vi "Alpha Ver 2.2.vi"() -> ()   [LabVIEW 2015]
uses:
  <instrlib>/Keithley 622x LV 2009/Keithley 622x.lvlib
  <instrlib>/Keithley 622x LV 2009/Utility/Typedefs/KE622x -- Instrument Type.ctl
panel:
  out "Measurements":string
  in  "Comments":string
  out "FILE":refnum<file>
  in  "Folder \nPrename":string
  out "Output command string":string
  out "Example of commands":string="*RST\nSOUR:PDEL:HIGH 1e-3\nSOUR:PDEL:LOW 0\nSOUR:PDEL:WIDT 500e-6\nSOUR:PDEL:SDEL 100e-6\nSOUR:PDEL:COUN INF\nSOUR:PDEL:RANG BEST\nSOUR:PDEL:INT 5\nSOUR:PDEL:LME 2\nTRAC:POIN 200\nSOUR:PDEL:ARM\nINIT:IMM"
  out "LM_com":string
  out "I_com":string
  out "R_com":string
  out "C_com":string
  out "SD_com":string
  out "W_com":string
  out "LL_com":string
  out "HL_com":string
  in  "INF Button":bool
  in  "prefix 2":u16(ring)
  in  "prefix":u16(ring)
  in  "Low Measure":u16(ring)=1 items=["1", "2"]
  in  "Interval":dbl=5.0 min=5.0 max=999999.0 step=1.0
  in  "Ranging":string(combo)="BEST"
  in  "Count":dbl=1.0 min=1.0 max=65536.0 step=1.0
  in  "Source Delay":dbl
  in  "Width":dbl
  in  "Low Level":dbl min=-0.105 max=0.105
  in  "High Level":dbl
  out "2182A \nconnected ?":string
  in  "STOP":bool
  out "Measurement\nUnits":string
  out "2182A Voltage \nRange":string
  out "error out":errorcluster
  # "Pulse Measurement System"
  # "SYSTEM INFORMATION"
  # "FILE CONFIGURATION"
  # "PULSE SETTINGS"
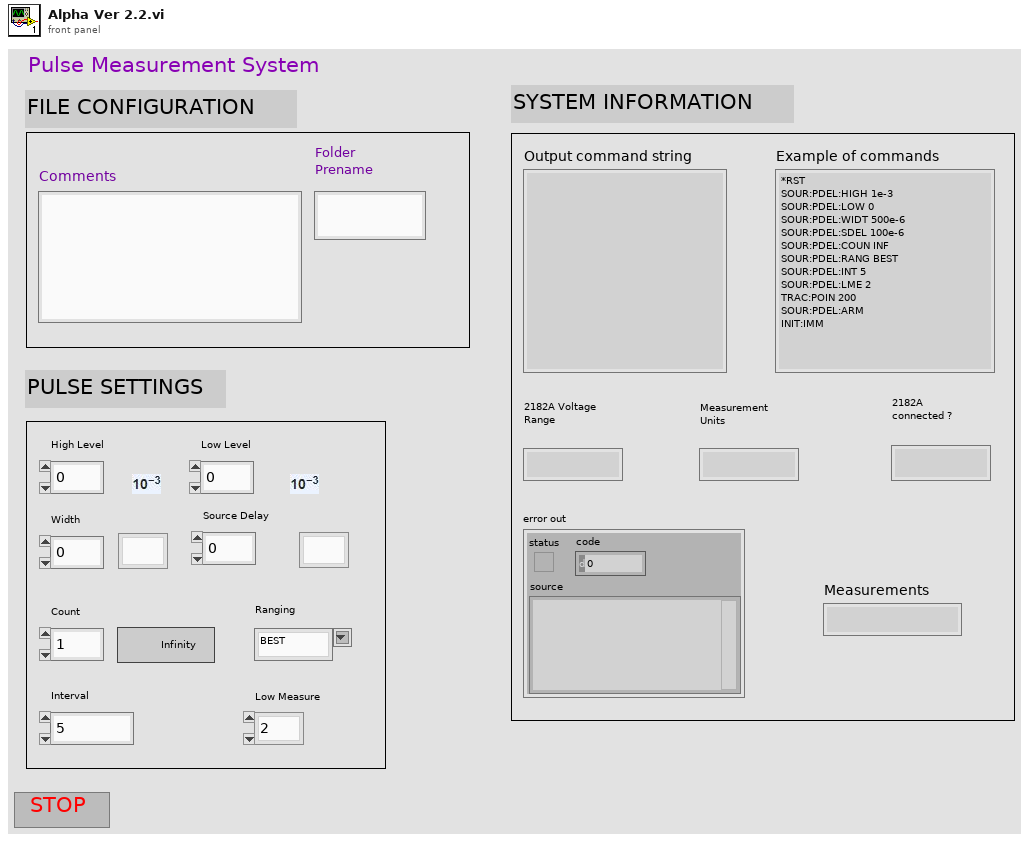
[diagram p1: front panel]
types:
  T1 = typedef "Keithley 622x.lvlib/KE622x -- Instrument Type.ctl" = enum16{"KE6220", "KE6221"}
  T2 = cluster{"VISA resource name out":refnum<visa-resource-name>, "error out":errorcluster}
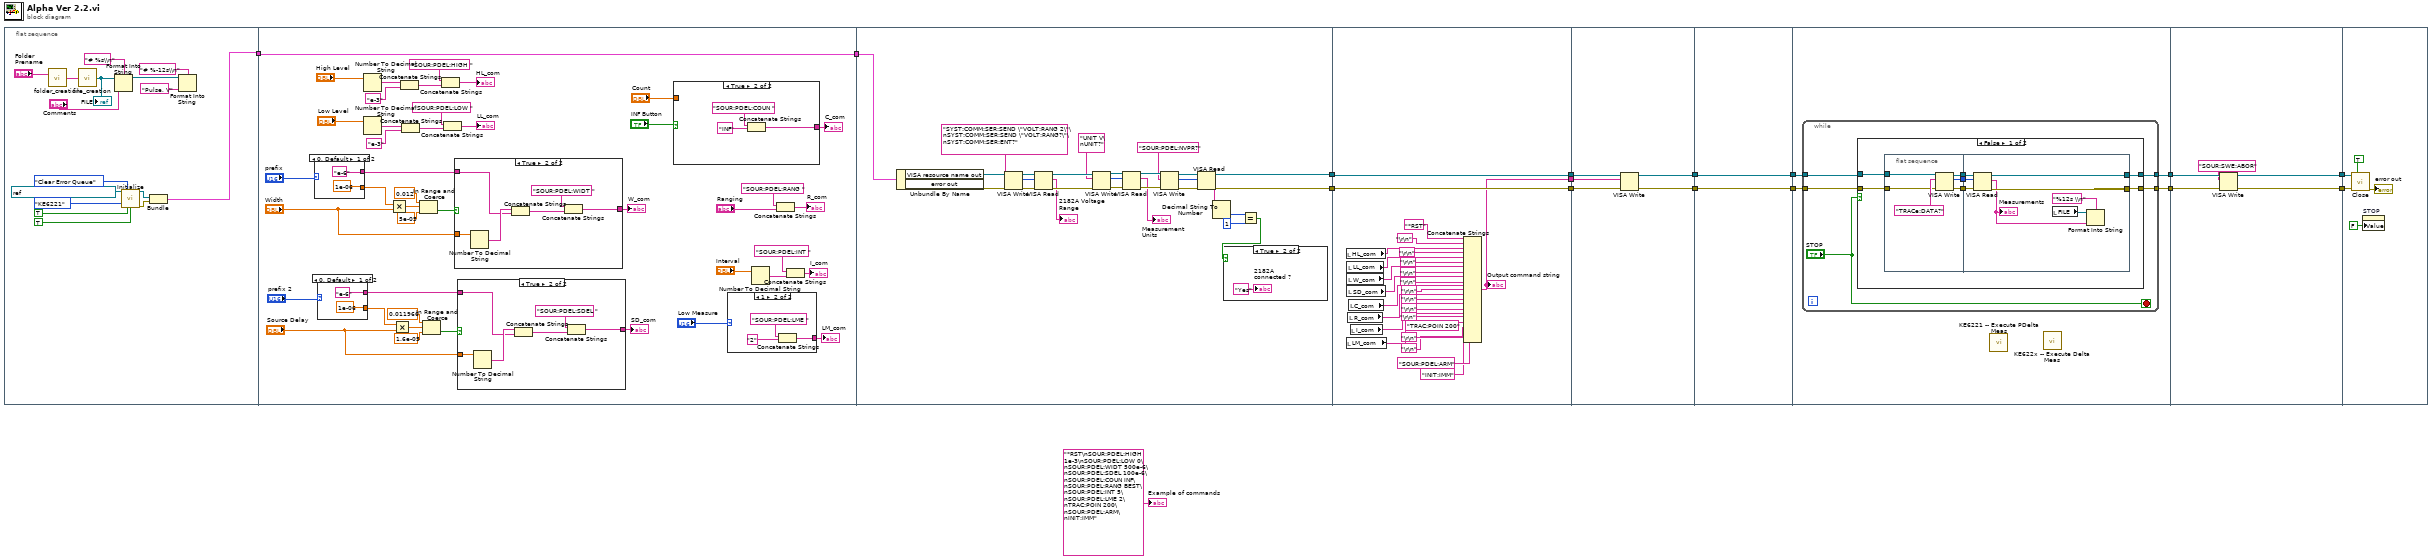
[diagram p0: block diagram]
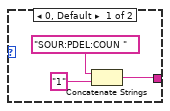
[diagram p2: hidden frame]
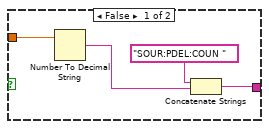
[diagram p3: hidden frame]
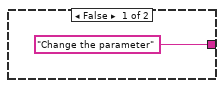
[diagram p4: hidden frame]
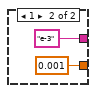
[diagram p5: hidden frame]
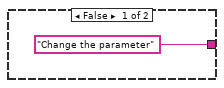
[diagram p6: hidden frame]
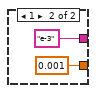
[diagram p7: hidden frame]
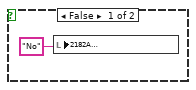
[diagram p8: hidden frame]
diagram:
  n1 = flat-sequence {
    tunnel: [w25] -> w16
    tunnel: w16 -> [w33]
    tunnel: [w33] -> w15
    tunnel: [w115] -> w14
    tunnel: [w114] -> w12
    tunnel: w15 -> [w113]
    tunnel: w14 -> [w165]
    tunnel: [w165] -> w13
    tunnel: w12 -> [w164]
    tunnel: [w164] -> w11
    tunnel: [w144] -> w9
    tunnel: w13 -> [w170]
    tunnel: [w169] -> w8
    tunnel: w11 -> [w168]
    tunnel: [w167] -> w6
    tunnel: w9 -> [w166]
    tunnel: w8 -> [w172]
    tunnel: [w172] -> w7
    tunnel: w6 -> [w171]
    tunnel: [w171] -> w5
    tunnel: w7 -> [w176]
    tunnel: w5 -> [w175]
    tunnel: [w174] -> w4
    tunnel: [w173] -> w2
    tunnel: w4 -> [w209]
    tunnel: [w208] -> w3
    tunnel: w2 -> [w207]
    tunnel: [w206] -> w1
    tunnel: w3 -> [w212]
    tunnel: w1 -> [w211]
    frame #0 {
      n2 = call "folder_creation.vi"("Name"="Folder \nPrename") -> ("String"=w23:string)
      n3 = call "file_creation.vi"("String"=w23) -> ("refnum out"=w22:refnum<file>)
      "FILE" <- w22
      n4 = Format Into String(format string="# %s\\n", initial string=w22, "Comments") -> (resulting string=w17:refnum<file>)  [unwired: 1 in, 1 out]
      n5 = call <instrlib>:"Initialize.vi"("VISA resource name"=refnum<visa-resource-name> "DC_AC_Current_Source_6221", "Error Queue Option"=enum16{"Clear Error Queue", "Error Query"}."Clear Error Queue", "Instrument Type"=KE622x_--_Instrument_Type."KE6221", "ID Query? (T)"=TRUE, "Reset? (T)"=TRUE) -> ("VISA resource name out"=w27:refnum<visa-resource-name>, "error out"=w26:errorcluster)  [unwired: 9 in]
      n6 = Bundle("VISA resource name out"=w27, "error out"=w26) -> (w25:T2)  [unwired: 1 in]
      n7 = Format Into String(format string="# %-12s\\n", initial string=w17, "Pulse, V" ("input 3")) -> ()  [unwired: 1 in, 2 out]
    }
    frame #1 {
      n8 = case shown="0, Default" "prefix" {
        tunnel: [1e-06 0.001] -> w56
        tunnel: ["e-6" ("string") "e-3" ("string")] -> w61
        frame 0, Default {
        }
        frame 1 {
        }
      }
      n9 = case shown="0, Default" "prefix 2" {
        tunnel: [1e-06 0.001] -> w51
        tunnel: ["e-6" ("string") "e-3" ("string")] -> w46
        frame 0, Default {
        }
        frame 1 {
        }
      }
      n10 = Number To Decimal String(number="High Level") -> (decimal integer string=w72:string)  [unwired: 1 in]
      n11 = Number To Decimal String(number="Low Level") -> (decimal integer string=w67:string)  [unwired: 1 in]
      n12 = Multiply(x=w56, y="Width") -> (x*y=w57:dbl)
      n13 = Multiply(x=w51, y="Source Delay") -> (x*y=w50:dbl)
      n14 = Concatenate Strings(w72, "e-3" ("string")) -> (w75:string)
      n15 = Concatenate Strings(w67, "e-3" ("string")) -> (w69:string)
      n16 = In Range and Coerce(upper limit=0.012, x=w57, lower limit=5e-05) -> (In Range?=w60:bool)  [unwired: 1 out]
      n17 = In Range and Coerce(upper limit=0.011966, x=w50, lower limit=1.6e-05) -> (In Range?=w47:bool)  [unwired: 1 out]
      n18 = Concatenate Strings("SOUR:PDEL:HIGH " ("string"), w75) -> (→"HL_com":string)
      n19 = Concatenate Strings("SOUR:PDEL:LOW " ("string"), w69) -> (→"LL_com":string)
      n20 = case shown="True" w60 {
        tunnel: w61 -> [_ w104]
        tunnel: "Width" -> [_ w106]
        tunnel: ["Change the parameter" w101] -> w63
        frame False {
        }
        frame True {
          n21 = Number To Decimal String(number=w106) -> (decimal integer string=w105:string)  [unwired: 1 in]
          n22 = Concatenate Strings(w105, w104) -> (w102:string)
          n23 = Concatenate Strings("SOUR:PDEL:WIDT " ("string"), w102) -> (w101:string)
        }
      }
      "W_com" <- w63
      n24 = case shown="True" w47 {
        tunnel: w46 -> [_ w93]
        tunnel: "Source Delay" -> [_ w95]
        tunnel: ["Change the parameter" w90] -> w54
        frame False {
        }
        frame True {
          n25 = Number To Decimal String(number=w95) -> (decimal integer string=w94:string)  [unwired: 1 in]
          n26 = Concatenate Strings(w94, w93) -> (w91:string)
          n27 = Concatenate Strings("SOUR:PDEL:SDEL " ("string"), w91) -> (w90:string)
        }
      }
      "SD_com" <- w54
      n28 = case shown="True" "INF Button" {
        tunnel: "Count" -> [w85 _]
        tunnel: [w83 w86] -> w45
        frame False {
          n29 = Number To Decimal String(number=w85) -> (decimal integer string=w82:string)  [unwired: 1 in]
          n30 = Concatenate Strings("SOUR:PDEL:COUN " ("string"), w82) -> (w83:string)
        }
        frame True {
          n31 = Concatenate Strings("SOUR:PDEL:COUN " ("string"), "INF") -> (w86:string)
        }
      }
      "C_com" <- w45
      n32 = case shown="1" "Low Measure" {
        tunnel: [w77 w79] -> w35
        frame 0, Default {
          n33 = Concatenate Strings("SOUR:PDEL:COUN " ("string"), "1" ("string")) -> (w77:string)
        }
        frame 1 {
          n34 = Concatenate Strings("SOUR:PDEL:LME " ("string"), "2") -> (w79:string)
        }
      }
      "LM_com" <- w35
      n35 = Number To Decimal String(number="Interval") -> (decimal integer string=w39:string)  [unwired: 1 in]
      n36 = Concatenate Strings("SOUR:PDEL:RANG " ("string"), "Ranging") -> (→"R_com":string)
      n37 = Concatenate Strings("SOUR:PDEL:INT " ("string"), w39) -> (→"I_com":string)
    }
    frame #2 {
      n38 = Unbundle By Name(w113) -> ("VISA resource name out"=w112:refnum<visa-resource-name>, "error out"=w111:errorcluster)
      n39 = VISA Write(VISA resource name=w112, write buffer="SYST:COMM:SER:SEND \"VOLT:RANG 2\"\nSYST:COMM:SER:SEND \"VOLT:RANG?\"\nSYST:COMM:SER:ENT?", error in (no error)=w111) -> (VISA resource name out=w135:refnum<visa-resource-name>, return count=w136:u32, error out=w134:errorcluster)
      n40 = VISA Read(VISA resource name=w135, byte count=w136, error in (no error)=w134) -> (VISA resource name out=w131:refnum<visa-resource-name>, read buffer=→"2182A Voltage \nRange":string, error out=w133:errorcluster)  [unwired: 1 out]
      n41 = VISA Write(VISA resource name=w131, write buffer="UNIT V\nUNIT?", error in (no error)=w133) -> (VISA resource name out=w127:refnum<visa-resource-name>, return count=w128:u32, error out=w129:errorcluster)
      n42 = VISA Read(VISA resource name=w127, byte count=w128, error in (no error)=w129) -> (VISA resource name out=w124:refnum<visa-resource-name>, read buffer=→"Measurement\nUnits":string, error out=w126:errorcluster)  [unwired: 1 out]
      n43 = VISA Write(VISA resource name=w124, write buffer="SOUR:PDEL:NVPR?", error in (no error)=w126) -> (VISA resource name out=w120:refnum<visa-resource-name>, return count=w121:u32, error out=w122:errorcluster)
      n44 = VISA Read(VISA resource name=w120, byte count=w121, error in (no error)=w122) -> (VISA resource name out=w115:refnum<visa-resource-name>, read buffer=w118:string, error out=w114:errorcluster)  [unwired: 1 out]
      n45 = Decimal String To Number(string=w118) -> (number=w117:i32)  [unwired: 2 in, 1 out]
      n46 = Equal?(x=w117, y=1) -> (x = y?=w119:bool)
      n47 = case shown="True" w119 {
        frame False {
          n48 = local write "2182A \nconnected ?"("No" ("2182A \nconnected ?")) -> ()
        }
        frame True {
          "2182A \nconnected ?" <- "Yes" ("2182A \nconnected ?")
        }
      }
    }
    frame #3 {
      n49 = local read "HL_com"() -> (w161:string)
      n50 = local read "LM_com"() -> (w147:string)
      n51 = local read "LL_com"() -> (w159:string)
      n52 = local read "W_com"() -> (w157:string)
      n53 = local read "SD_com"() -> (w155:string)
      n54 = local read "R_com"() -> (w152:string)
      n55 = local read "C_com"() -> (w153:string)
      n56 = local read "I_com"() -> (w149:string)
      n57 = Concatenate Strings("*RST" ("string"), "\r\n", w161, "\r\n", w159, "\r\n", w157, "\r\n", w155, "\r\n", w153, "\r\n", w152, "\r\n", w149, "\r\n", w147, "\r\n", "TRAC:POIN 200" ("string"), "\r\n", "SOUR:PDEL:ARM" ("string"), "\r\n", "INIT:IMM" ("string")) -> (w144:string)
      "Output command string" <- w144
    }
    frame #4 {
      n58 = VISA Write(VISA resource name=w170, write buffer=w166, error in (no error)=w168) -> (VISA resource name out=w169:refnum<visa-resource-name>, error out=w167:errorcluster)  [unwired: 1 out]
    }
    frame #5 {
    }
    frame #6 {
      n59 = while {
        tunnel: w176 -> [w181]
        tunnel: w175 -> [w180]
        tunnel: [w178] -> w174
        tunnel: [w177] -> w173
        stop <- "STOP" stop-if-true
        n60 = case shown="False" "STOP" {
          tunnel: w181 -> [w188 w204]
          tunnel: w180 -> [w187 w203]
          tunnel: [w182 w204] -> w178
          tunnel: [w183 w203] -> w177
          frame False {
            n61 = flat-sequence {
              tunnel: w188 -> [w193]
              tunnel: w187 -> [w192]
              tunnel: [w191] -> w186
              tunnel: [w190] -> w185
              tunnel: [w189] -> w184
              tunnel: w186 -> [w202]
              tunnel: w185 -> [w201]
              tunnel: w184 -> [w200]
              tunnel: [w199] -> w183
              tunnel: [w198] -> w182
              frame #0 {
                n62 = VISA Write(VISA resource name=w193, write buffer="TRACe:DATA?", error in (no error)=w192) -> (VISA resource name out=w191:refnum<visa-resource-name>, return count=w189:u32, error out=w190:errorcluster)
              }
              frame #1 {
                n63 = VISA Read(VISA resource name=w202, byte count=w200, error in (no error)=w201) -> (VISA resource name out=w198:refnum<visa-resource-name>, read buffer=w196:string, error out=w199:errorcluster)  [unwired: 1 out]
                "Measurements" <- w196
                n64 = local read "FILE"() -> (w195:refnum<file>)
                n65 = Format Into String(format string="%12s \\n", initial string=w195, w196) -> ()  [unwired: 1 in, 2 out]
              }
            }
          }
          frame True {
          }
        }
      }
      n66 = call <instrlib>:"KE6221 -- Execute PDelta Meas.vi"() -> ()  [unwired: 10 in, 6 out]
      n67 = call <instrlib>:"KE622x -- Execute Delta Meas.vi"() -> ()  [unwired: 10 in, 6 out]
    }
    frame #7 {
      n68 = VISA Write(VISA resource name=w209, write buffer="SOUR:SWE:ABOR", error in (no error)=w207) -> (VISA resource name out=w208:refnum<visa-resource-name>, error out=w206:errorcluster)  [unwired: 1 out]
    }
    frame #8 {
      n69 = call <instrlib>:"Close.vi"("VISA resource name"=w212, "Query For SCPI Errors? (T)"=TRUE, "error in (no error)"=w211) -> ("error out"=→"error out":errorcluster)  [unwired: 12 in]
      n70 = property on="STOP" class="Bool (strict)"("Value"=FALSE ("STOP")) -> ()  [unwired: 2 in, 2 out]
    }
  }
  "Example of commands" <- "*RST\nSOUR:PDEL:HIGH 1e-3\nSOUR:PDEL:LOW 0\nSOUR:PDEL:WIDT 500e-6\nSOUR:PDEL:SDEL 100e-6\nSOUR:PDEL:COUN INF\nSOUR:PDEL:RANG BEST\nSOUR:PDEL:INT 5\nSOUR:PDEL:LME 2\nTRAC:POIN 200\nSOUR:PDEL:ARM\nINIT:IMM" ("write buffer")
